vi "test - #86.vi"(8 "error in (no error)":errorcluster, 11 "TestCase in":refnum<class "testcase-Supported-Datatype.lvclass">) -> (0 "error out":errorcluster, 3 "TestCase out":refnum<class "testcase-Supported-Datatype.lvclass">)   [LabVIEW 2017, in "testcase-Supported-Datatype.lvclass"]
uses:
  testcase-Supported-Datatype.lvclass
  aa1c4cdf-b71f-44fa-881a-9758266639fc.vi
  422887b0-169e-41e8-b0db-8320d9243545.vi
  addons/API-String-Arugments-Support/_Support/Data To API String Arguments.vi
  addons/API-String-Arugments-Support/_Support/Convert API String Arguments to Data(variant).vi
  <vilib>/addons/_JKI Toolkits/VI Tester/TestCase.llb/TestCase.lvclass
  C:/Program Files (x86)/National Instruments/LabVIEW 2017/vi.lib/addons/_JKI Toolkits/VI Tester/TestCase.llb/TestCase.lvclass
panel:
  out "String":string
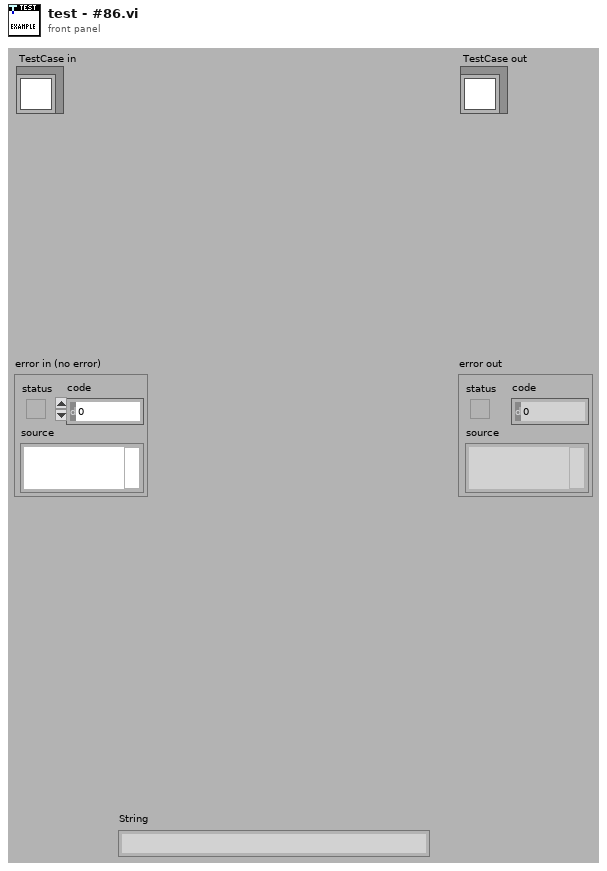
[diagram p1: front panel]
types:
  T1 = cluster{"1":bool, "2":i32[], "3":cluster{"3.1":string, "3.2":dbl, "3.3":bool}, "5":cluster{"5.2":bool}}
  T2 = cluster{"6":string, "1":bool, "5":cluster{"5.1":string[], "5.2":bool}, "2":i32[], "3":cluster{"3.1":string, "3.2":dbl, "3.3":bool, "3.4":i32[]}, "4":path}
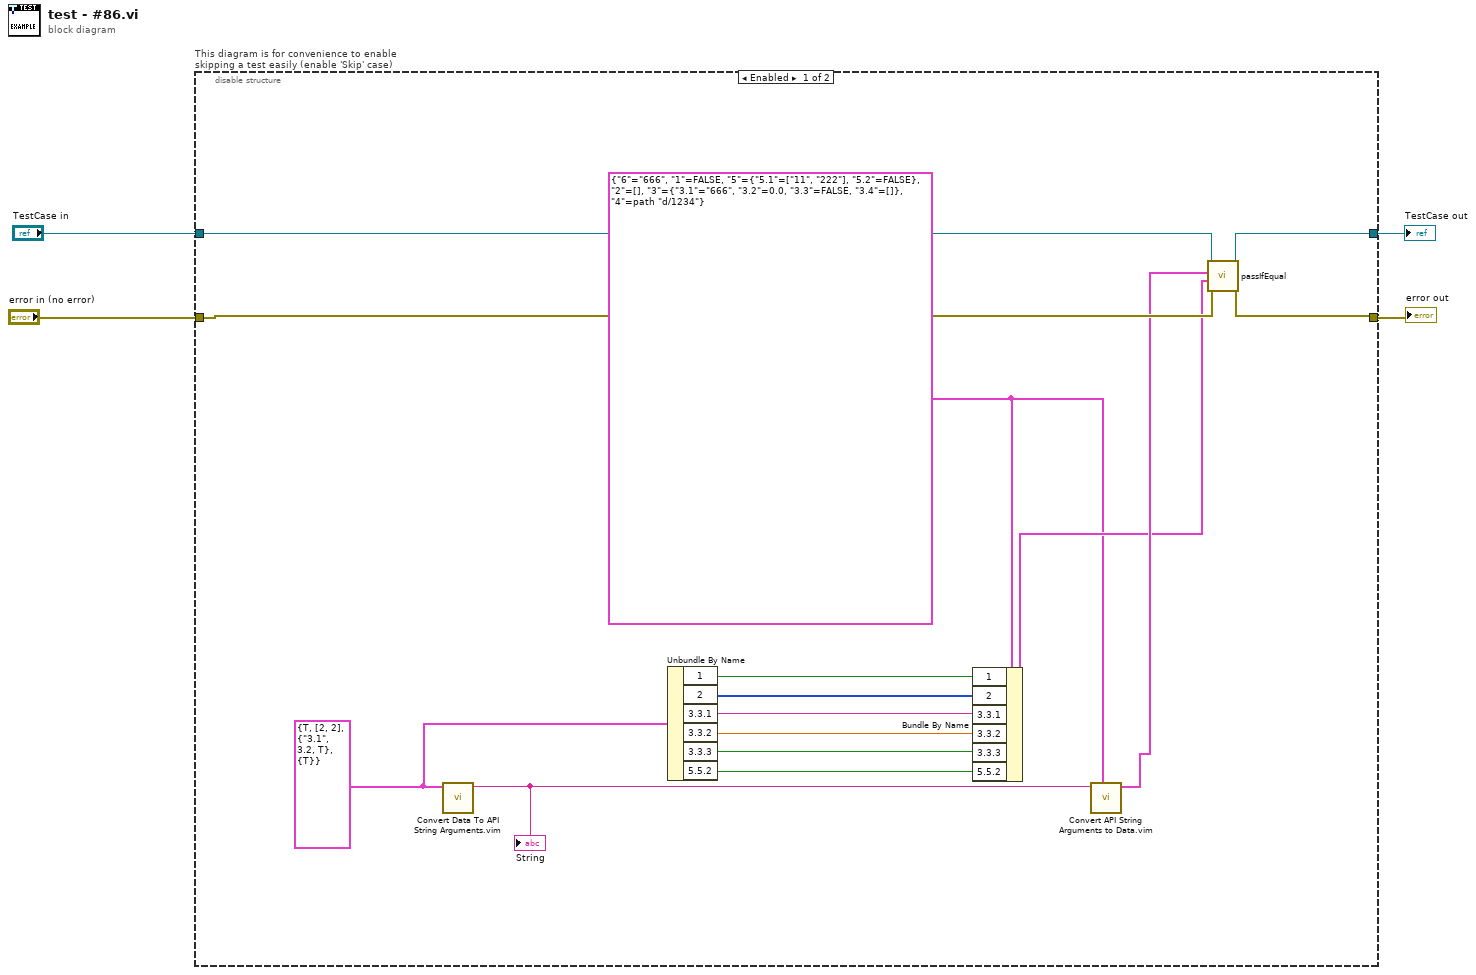
[diagram p0: block diagram]
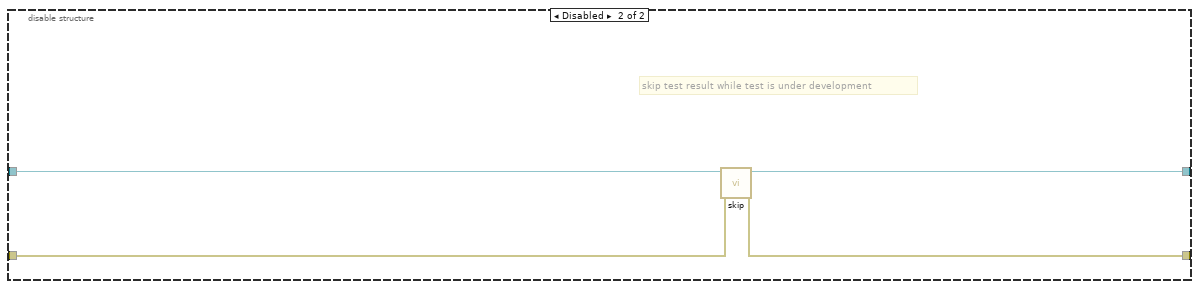
[diagram p2: hidden frame]
diagram:
  n1 = disable-structure "This diagram is for convenience to enable skipping a test easily (enable 'Skip' case)" shown="Enabled" {
    disable-tunnel: "TestCase in" -> [w19 w23]
    disable-tunnel: [w18 w21] -> w1
    disable-tunnel: [w17 w22] -> w3
    disable-tunnel: "error in (no error)" -> [w16 w20]
    frame Enabled {
      w13 = T1 {"1"=TRUE, "2"=[2, 2], "3"={"3.1"="3.1", "3.2"=3.2, "3.3"=TRUE}, "5"={"5.2"=TRUE}} ("Cluster")
      w5 = T2 {"6"="666", "1"=FALSE, "5"={"5.1"=["11", "222"], "5.2"=FALSE}, "2"=[], "3"={"3.1"="666", "3.2"=0.0, "3.3"=FALSE, "3.4"=[]}, "4"=path "d:/1234"}
      n2 = call "Convert Data To API String Arguments.vim"("Data"=w13) -> ("API String"=w15:string)  [unwired: 7 in, 1 out]
      "String" <- w15
      n3 = Unbundle By Name(w13) -> ("1"=w12:bool, "2"=w7:i32[], "3.3.1"=w8:string, "3.3.2"=w9:dbl, "3.3.3"=w10:bool, "5.5.2"=w11:bool)
      n4 = Bundle By Name(cluster=w5, "1"=w12, "2"=w7, "3.3.1"=w8, "3.3.2"=w9, "3.3.3"=w10, "5.5.2"=w11) -> (w6:T2)
      n5 = call "Convert API String Arguments to Data.vim"("Reference Type"=w5, "API String"=w15) -> ("Data"=w14:T2)  [unwired: 6 in, 1 out]
      n6 = call-dynamic "passIfEqual.vi"("error in (no error)"=w16, "y"=w6, "x"=w14, "TestCase in"=w19) -> ("error out"=w17:errorcluster, "TestCase out"=w18:refnum<class "testcase-Supported-Datatype.lvclass">)  [unwired: 6 in]
    }
    frame Disabled {
      # "skip test result while test is under development"
      n7 = call <vilib>:"skip.vi"("error in (no error)"=w20, "TestCase in"=w23) -> ("error out"=w22:errorcluster, "TestCase out"=w21:refnum<class "testcase-Supported-Datatype.lvclass">)  [unwired: 8 in]
    }
  }
  "error out" <- w3
  "TestCase out" <- w1
